vi "Write Values.vi"(8 "error in (no error)":errorcluster, 9 "Sentence Index":i32, 10 "Values":dbl[](array[numeric]), 11 "Multi Parser in":refnum<class "Multi Sentence Parser.lvclass">) -> (0 "error out":errorcluster, 3 "Multi Parser out":refnum<class "Multi Sentence Parser.lvclass">)   [LabVIEW 2024, in "Multi Sentence Parser.lvclass"]
doc: "Multi Sentence Parser.lvclass:Write Values.vi\n\nThis VI writes the values for one sentence into the class data memory.\n\nInstrument Communication Module Version 1.0\nOctober, 2018 Original Code Consulting David Thomson\n www.originalcode.com"
uses:
  Multi Sentence Parser.lvclass
  Multi Sentence Parser.lvclass/Multi Sentence Parser.ctl
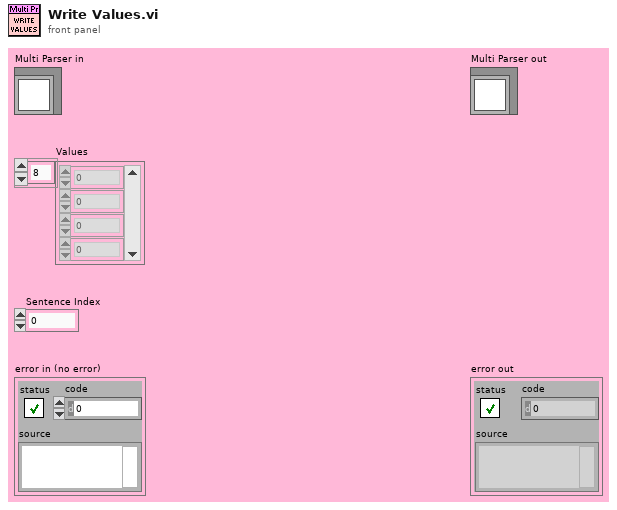
[diagram p1: front panel]
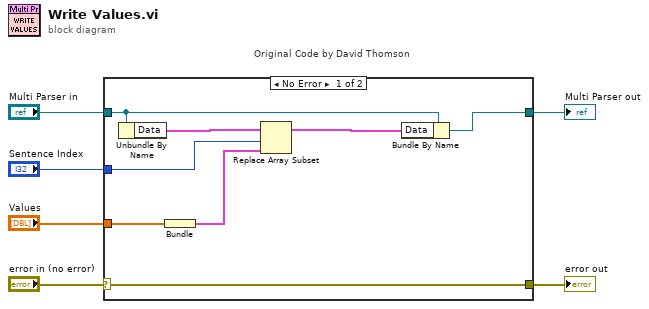
[diagram p0: block diagram]
diagram:
  n1 = case "Original Code by David Thomson" shown="No Error" "error in (no error)" {
    selector: "error in (no error)" -> [w14 w15]
    tunnel: [w14 w15] -> w5
    tunnel: [w8 w16] -> w3
    tunnel: "Multi Parser in" -> [w9 w16]
    tunnel: "Values" -> [w11 _]
    tunnel: "Sentence Index" -> [w10 _]
    frame No Error {
      n2 = Unbundle By Name(w9) -> ("Data"=w13:cluster{"1 Sentence":dbl[]}[])
      n3 = Bundle("Values"=w11) -> (w12:cluster{"Values":dbl[]})  [unwired: 1 in]
      n4 = Replace Array Subset(array=w13, new element=w12, index=w10) -> (w7:cluster{"1 Sentence":dbl[]}[])
      n5 = Bundle By Name(cluster=w9, "Data"=w7) -> (w8:refnum<class "Multi Sentence Parser.lvclass">)
    }
    frame Error {
    }
  }
  "error out" <- w5
  "Multi Parser out" <- w3
